vi "Temp_controller_with_cooling.vi"() -> ()   [LabVIEW 2017]
uses:
  <instrlib>/Lake Shore Cryotronics 332/Lake Shore Cryotronics 332.lvlib
panel:
  out "error out 2":errorcluster
  out "error out":errorcluster
  in  "Rate(D)":dbl min=0.0 max=200.0 step=1.0
  in  "Reset (I) (0.0)":dbl min=0.0 max=1000.0 step=0.1 format="%.1f"
  in  "Gain (P)":dbl min=0.0 max=1000.0 step=0.1 format="%.1f"
  in  "Manual Output":dbl min=0.0 max=100.0 step=0.001 format="%.3f"
  in  "Heater Range ()":u16(ring) items=["Off", "Low (0.5W)", "Med (5W)", "High (50W)"]
  out "Gain (P) 2":dbl min=0.0 max=1000.0 step=0.1 format="%.1f"
  out "Reset (I)":dbl min=0.0 max=1000.0 step=0.1 format="%.1f"
  out "Rate (D)":dbl min=0.0 max=1000.0 step=0.1 format="%.1f"
  out "Loop 1 Heater Range":u16(ring) items=["Off", "Low (0.5W)", "Med (5W)", "High (50W)"]
  in  "Enable Powerup ()":bool
  in  "Control Mode":u16(ring) items=["Manual PID", "Zone", "Open Loop", "AutoTune PID", "AutoTune PI", "AutoTune P"]
  out "return count 2":u32
  out "?":u32
  in  "error in (no error) 2":errorcluster
  in  "VISA resource name":refnum<visa-resource-name>
  in  "time interval to wait":dbl
  out "return count":u32
  out "?":u32
  in  "error in (no error)":errorcluster
  in  "Temo diff":dbl
  in  "End Temp":dbl
  in  "Start Temp":dbl
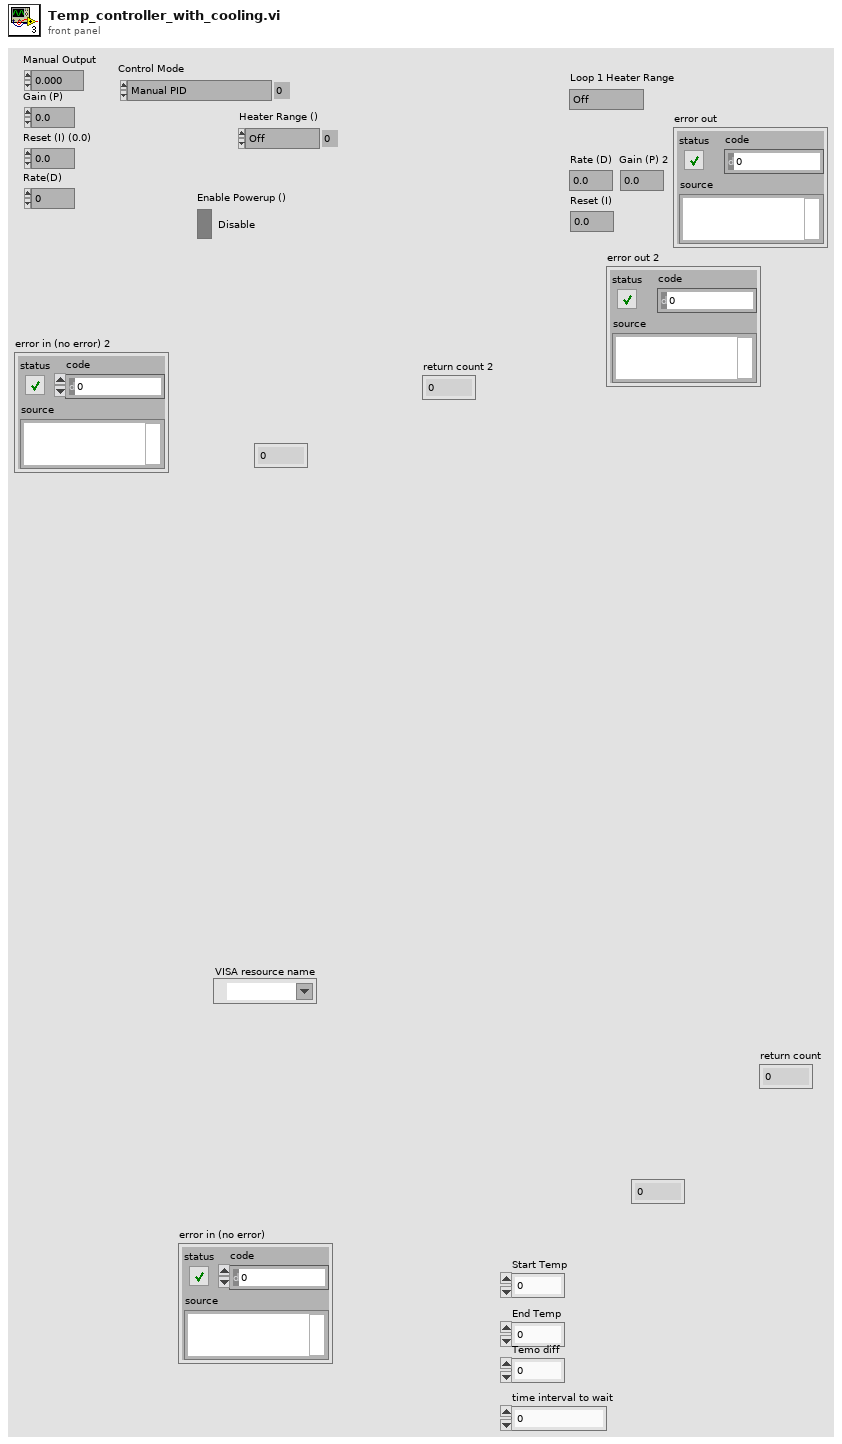
[diagram p1: front panel]
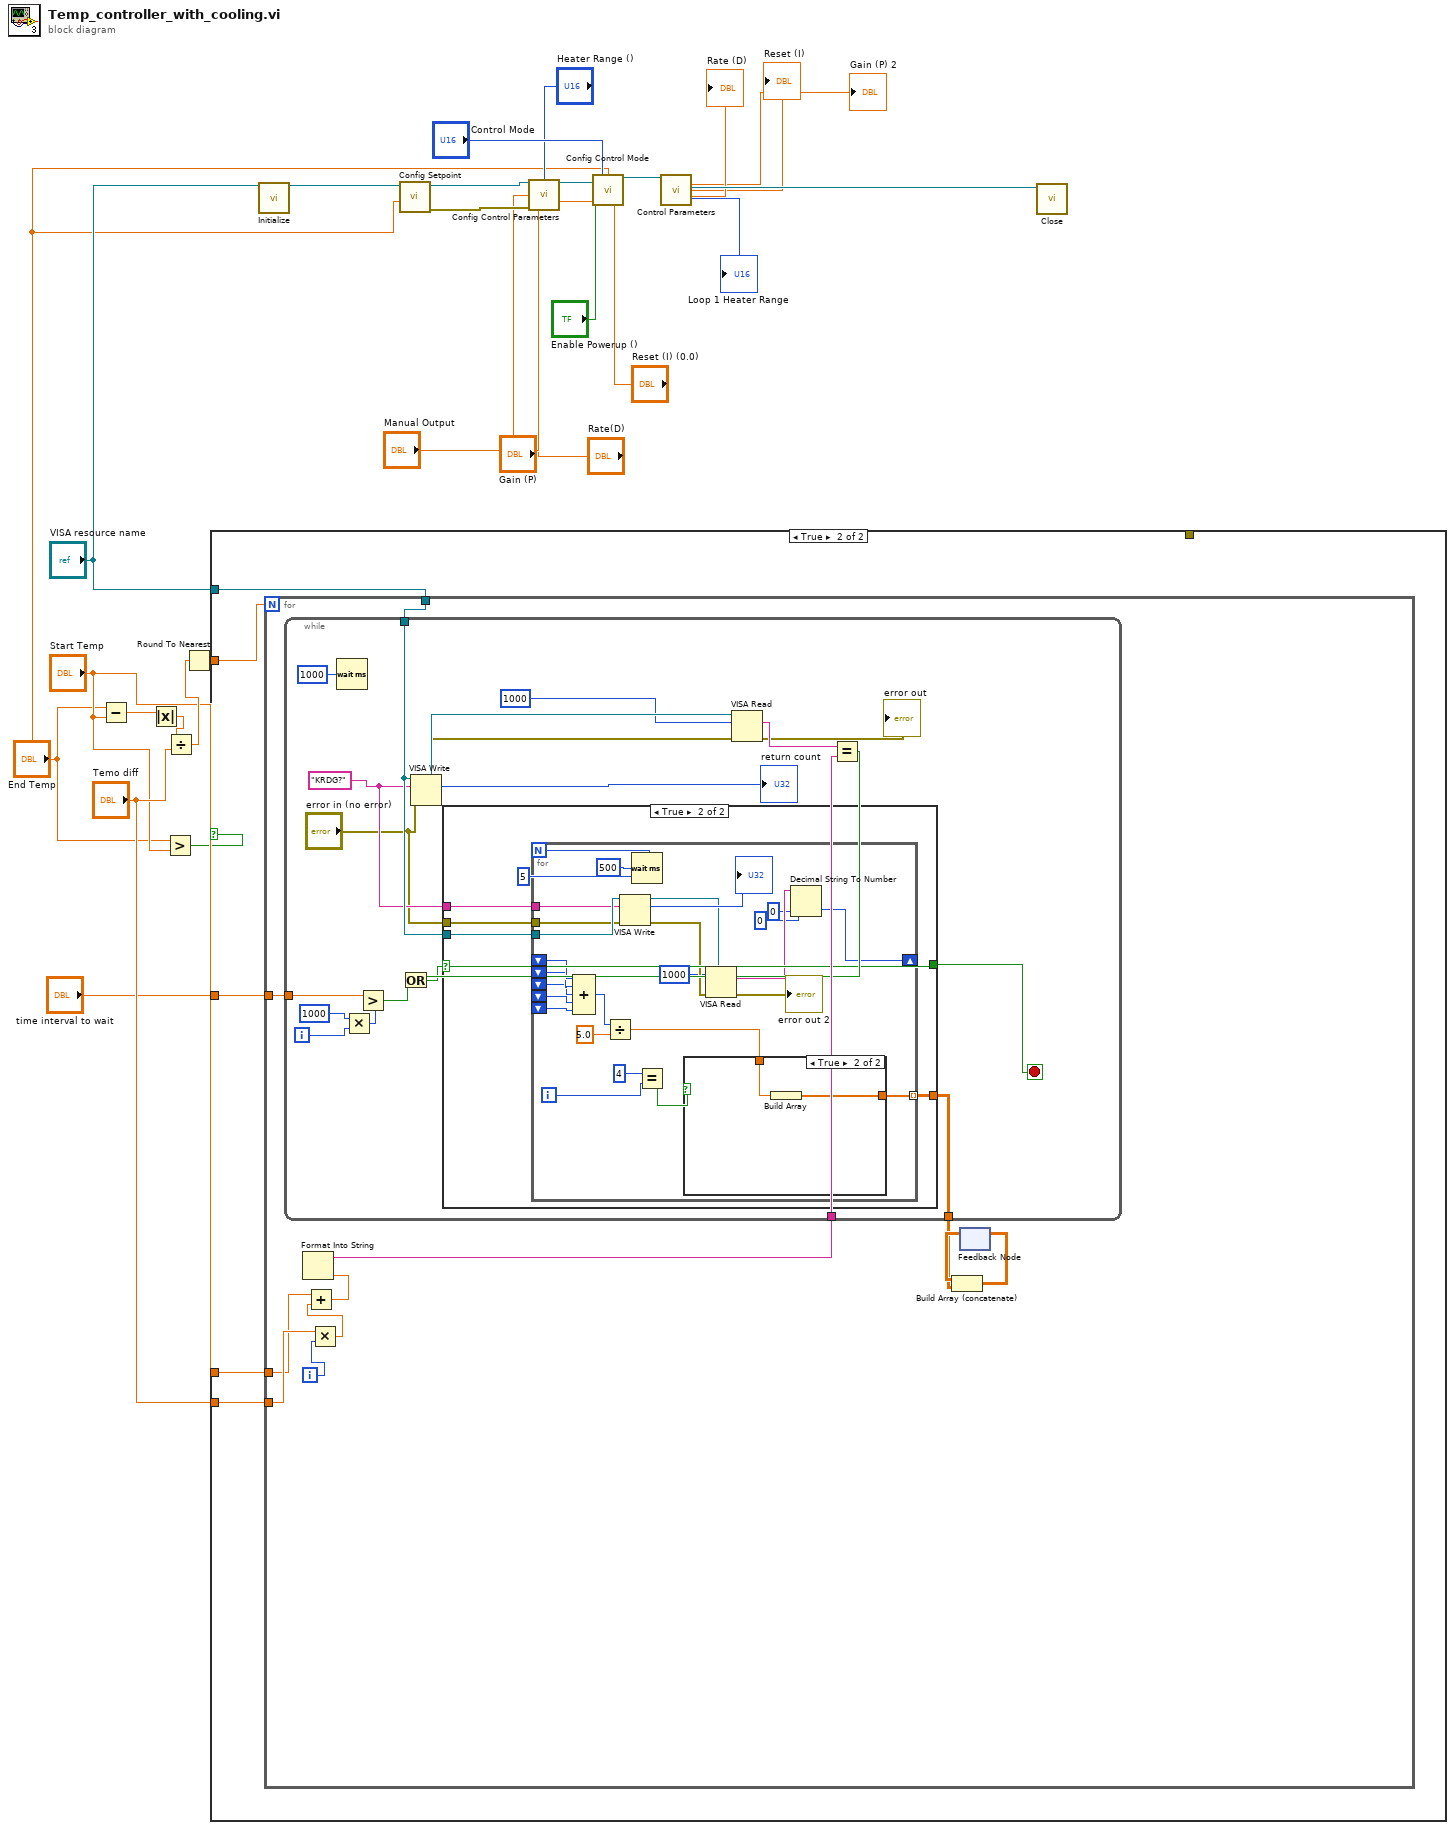
[diagram p0: block diagram]
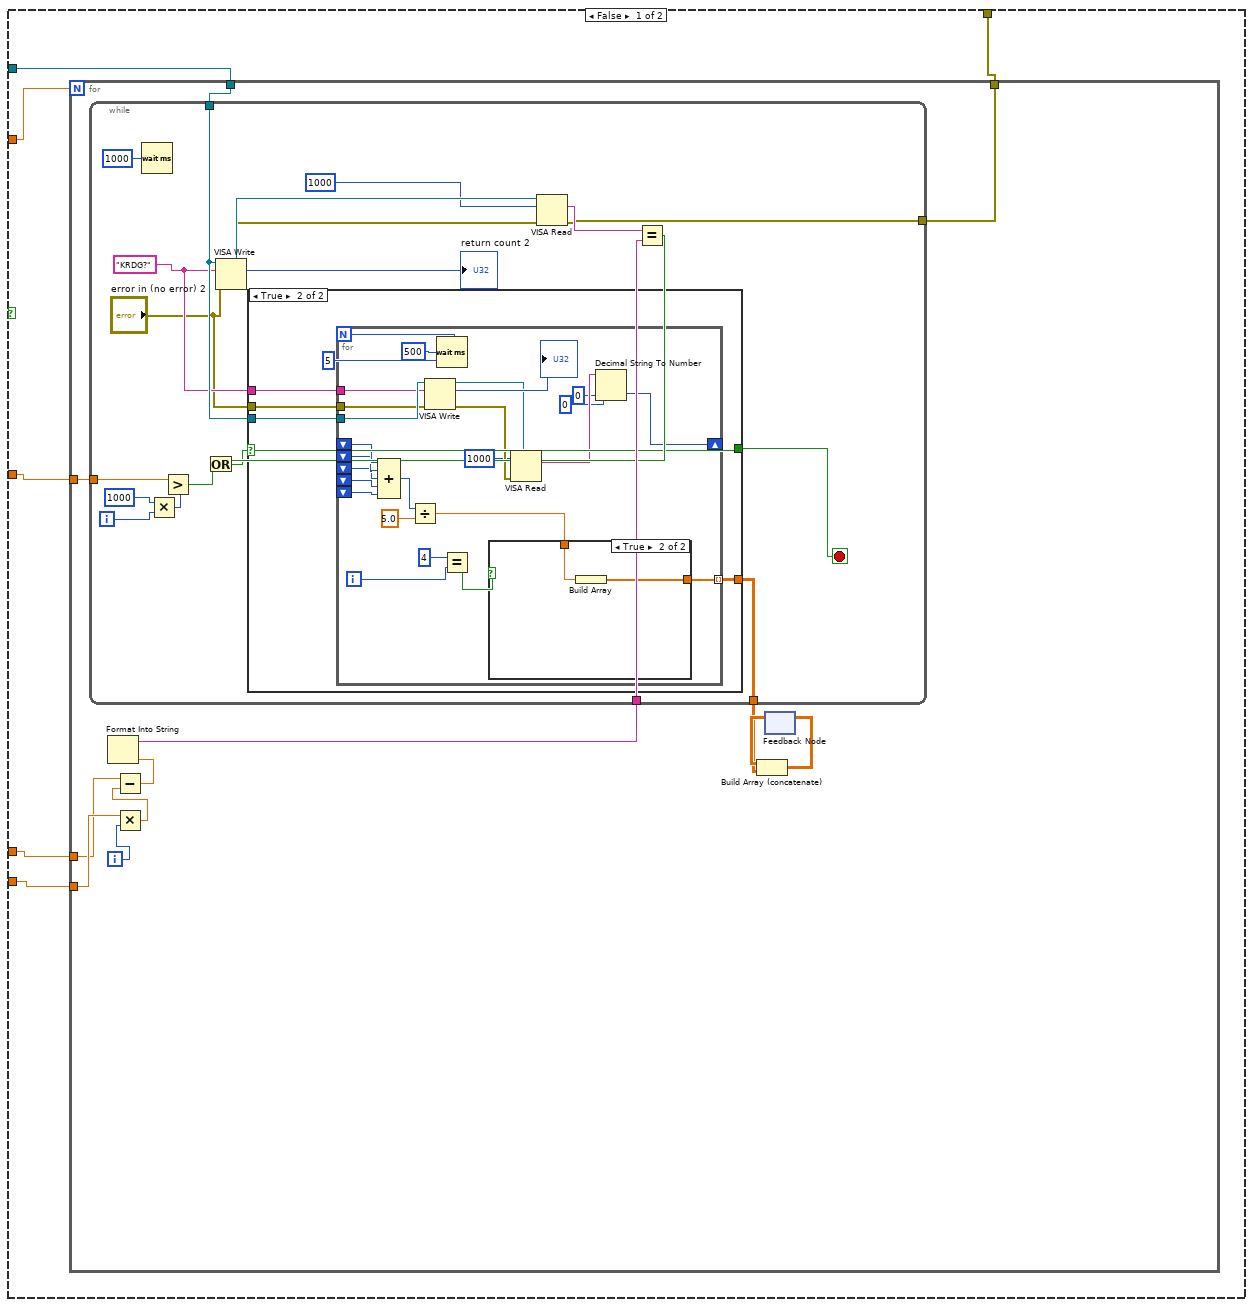
[diagram p2: hidden frame]
diagram:
  n1 = Subtract(x="End Temp", y="Start Temp") -> (x-y=w21:dbl)
  n2 = Absolute Value(x=w21) -> (abs(x)=w20:dbl)
  n3 = Greater?(x="End Temp", y="Start Temp") -> (0:w22:bool)
  n4 = Divide(x=w20, y="Temo diff") -> (x/y=w27:dbl)
  n5 = Round To Nearest(number=w27) -> (nearest integer value=w26:dbl)
  n6 = case shown="True" w22 {
    tunnel: w26 -> [w32 w103]
    tunnel: "Temo diff" -> [w28 w102]
    tunnel: "Start Temp" -> [w29 w101]
    tunnel: "VISA resource name" -> [w33 w100]
    tunnel: "time interval to wait" -> [w31 w99]
    tunnel: [w30 _] -> _
    frame False {
      n7 = for {
        N: w32 -> [_]
        tunnel: w28 -> [w45]
        tunnel: w29 -> [w36]
        tunnel: w33 -> [w44]
        tunnel: w31 -> [w43]
        tunnel: [w37] -> w30
        i -> [w42]
        n8 = Multiply(x=w45, y=w42) -> (x*y=w35:dbl)
        n9 = Subtract(x=w36, y=w35) -> (x-y=w34:dbl)
        n10 = Format Into String(w34) -> (resulting string=w41:string)  [unwired: 3 in, 1 out]
        n11 = while {
          tunnel: w44 -> [w54]
          tunnel: w41 -> [w60]
          tunnel: w43 -> [w55]
          tunnel: [w51] -> w38
          tunnel: [w46] -> w37
          i -> [w58]
          stop <- w48 stop-if-true
          w52 = "KRDG?" ("write buffer")
          n12 = Wait (ms)(milliseconds to wait=u32 1000) -> ()  [unwired: 1 out]
          n13 = Multiply(x=1000, y=w58) -> (x*y=w56:i32)
          n14 = Greater?(x=w55, y=w56) -> (0:w53:bool)
          n15 = VISA Write(VISA resource name=w54, write buffer=w52, error in (no error)="error in (no error) 2") -> (VISA resource name out=w64:refnum<visa-resource-name>, return count=→"return count 2":u32, error out=w62:errorcluster)
          n16 = VISA Read(VISA resource name=w64, byte count=u32 1000, error in (no error)=w62) -> (read buffer=w59:string, error out=w46:errorcluster)  [unwired: 2 out]
          n17 = Equal?(x=w59, y=w60) -> (x = y?=w50:bool)
          n18 = Or(x=w50, y=w53) -> (x .or. y?=w49:bool)
          n19 = case shown="True" w49 {
            selector: w49 -> [w66 w68]
            tunnel: w54 -> [_ w71]
            tunnel: w52 -> [_ w70]
            tunnel: [_ w69] -> w51
            tunnel: [w66 w68] -> w48
            tunnel: "error in (no error) 2" -> [_ w67]
            frame False {
            }
            frame True {
              n20 = for {
                N: 5 -> [_]
                tunnel: w71 -> [w93]
                shift-right: [w87] -> _
                shift-left: _ -> [w86]
                shift-left: _ -> [w85]
                shift-left: _ -> [w84]
                shift-left: _ -> [w83]
                shift-left: _ -> [w82]
                tunnel: w70 -> [w77]
                tunnel: [w75] -> w69 mode=indexing
                tunnel: w67 -> [w73]
                i -> [w79]
                n21 = Compound Arithmetic op=ADD(w86, w85, w84, w83, w82) -> (w80:i32)
                n22 = Divide(x=w80, y=5.0) -> (x/y=w76:dbl)
                n23 = VISA Write(VISA resource name=w93, write buffer=w77, error in (no error)=w73) -> (VISA resource name out=w92:refnum<visa-resource-name>, return count=→"?":u32, error out=w95:errorcluster)
                n24 = Wait (ms)(milliseconds to wait=u32 500) -> ()  [unwired: 1 out]
                n25 = Equal?(x=4, y=w79) -> (x = y?=w74:bool)
                n26 = case shown="True" w74 {
                  tunnel: w76 -> [_ w98]
                  tunnel: [_ w97] -> w75
                  frame False {
                  }
                  frame True {
                    n27 = Build Array(w98) -> (w97:dbl[])
                  }
                }
                n28 = VISA Read(VISA resource name=w92, byte count=u32 1000, error in (no error)=w95) -> (read buffer=w90:string)  [unwired: 3 out]
                n29 = Decimal String To Number(string=w90, offset=0, default (0L)=0 ("default (0 I32)")) -> (number=w87:i32)  [unwired: 1 out]
              }
            }
          }
        }
        n30 = feedback #1() -> (w39:dbl[][][])  [unwired: 1 in]
        n31 = Build Array (concatenate)(w39, w38) -> (w40:dbl[][][])
        n32 = feedback-in #1(w40) -> ()
      }
    }
    frame True {
      n33 = for {
        N: w103 -> [_]
        tunnel: w102 -> [w114]
        tunnel: w101 -> [w113]
        tunnel: w100 -> [w110]
        tunnel: w99 -> [w109]
        i -> [w108]
        n34 = Multiply(x=w114, y=w108) -> (x*y=w112:dbl)
        n35 = Add(x=w113, y=w112) -> (x+y=w111:dbl)
        n36 = Format Into String(w111) -> (resulting string=w107:string)  [unwired: 3 in, 1 out]
        n37 = while {
          tunnel: w110 -> [w123]
          tunnel: w107 -> [w129]
          tunnel: w109 -> [w124]
          tunnel: [w120] -> w104
          i -> [w127]
          stop <- w117 stop-if-true
          w121 = "KRDG?" ("write buffer")
          n38 = Wait (ms)(milliseconds to wait=u32 1000) -> ()  [unwired: 1 out]
          n39 = Multiply(x=1000, y=w127) -> (x*y=w125:i32)
          n40 = Greater?(x=w124, y=w125) -> (0:w122:bool)
          n41 = VISA Write(VISA resource name=w123, write buffer=w121, error in (no error)="error in (no error)") -> (VISA resource name out=w133:refnum<visa-resource-name>, return count=→"return count":u32, error out=w131:errorcluster)
          n42 = VISA Read(VISA resource name=w133, byte count=u32 1000, error in (no error)=w131) -> (read buffer=w128:string, error out=→"error out":errorcluster)  [unwired: 2 out]
          n43 = Equal?(x=w128, y=w129) -> (x = y?=w119:bool)
          n44 = Or(x=w119, y=w122) -> (x .or. y?=w118:bool)
          n45 = case shown="True" w118 {
            selector: w118 -> [w135 w137]
            tunnel: w123 -> [_ w140]
            tunnel: w121 -> [_ w139]
            tunnel: [_ w138] -> w120
            tunnel: [w135 w137] -> w117
            tunnel: "error in (no error)" -> [_ w136]
            frame False {
            }
            frame True {
              n46 = for {
                N: 5 -> [_]
                tunnel: w140 -> [w163]
                shift-right: [w157] -> _
                shift-left: _ -> [w156]
                shift-left: _ -> [w155]
                shift-left: _ -> [w154]
                shift-left: _ -> [w153]
                shift-left: _ -> [w152]
                tunnel: w139 -> [w147]
                tunnel: [w145] -> w138 mode=indexing
                tunnel: w136 -> [w143]
                i -> [w149]
                n47 = Compound Arithmetic op=ADD(w156, w155, w154, w153, w152) -> (w150:i32)
                n48 = Divide(x=w150, y=5.0) -> (x/y=w146:dbl)
                n49 = VISA Write(VISA resource name=w163, write buffer=w147, error in (no error)=w143) -> (VISA resource name out=w162:refnum<visa-resource-name>, return count=→"?":u32, error out=w165:errorcluster)
                n50 = Wait (ms)(milliseconds to wait=u32 500) -> ()  [unwired: 1 out]
                n51 = Equal?(x=4, y=w149) -> (x = y?=w144:bool)
                n52 = case shown="True" w144 {
                  tunnel: w146 -> [_ w168]
                  tunnel: [_ w167] -> w145
                  frame False {
                  }
                  frame True {
                    n53 = Build Array(w168) -> (w167:dbl[])
                  }
                }
                n54 = VISA Read(VISA resource name=w162, byte count=u32 1000, error in (no error)=w165) -> (read buffer=w160:string, error out=→"error out 2":errorcluster)  [unwired: 2 out]
                n55 = Decimal String To Number(string=w160, offset=0, default (0L)=0 ("default (0 I32)")) -> (number=w157:i32)  [unwired: 1 out]
              }
            }
          }
        }
        n56 = feedback #2() -> (w105:dbl[][][])  [unwired: 1 in]
        n57 = Build Array (concatenate)(w105, w104) -> (w106:dbl[][][])
        n58 = feedback-in #2(w106) -> ()
      }
    }
  }
  n59 = call <instrlib>:"Initialize.vi"("VISA resource name"="VISA resource name") -> ("VISA resource name out"=w19:refnum<visa-resource-name>)  [unwired: 13 in, 1 out]
  n60 = call <instrlib>:"Config Setpoint.vi"("Setpoint (0.0000)"="End Temp", "VISA resource name"=w19) -> ("error out"=w10:errorcluster, "VISA resource name out"=w11:refnum<visa-resource-name>)  [unwired: 8 in]
  n61 = call <instrlib>:"Config Control Parameters.vi"("VISA resource name"=w11, "Manual Output (0.000)"="Manual Output", "Heater Range (0: Off)"="Heater Range ()", "Gain (P) (0.0)"="Gain (P)", "Reset (I) (0.0)"="Reset (I) (0.0)", "error in (no error)"=w10, "Rate (D) (0)"="Rate(D)") -> ("VISA resource name out"=w9:refnum<visa-resource-name>)  [unwired: 7 in, 1 out]
  n62 = call <instrlib>:"Config Control Mode.vi"("VISA resource name"=w9, "Control Mode (0: Manual PID)"="Control Mode", "Setpoint Units (0: Kelvin)"="End Temp", "Enable Powerup (F: Enable)"="Enable Powerup ()") -> ("VISA resource name out"=w3:refnum<visa-resource-name>)  [unwired: 10 in, 1 out]
  n63 = call <instrlib>:"Control Parameters.vi"("VISA resource name"=w3) -> ("VISA resource name out"=w18:refnum<visa-resource-name>, "Gain (P)"=→"Gain (P) 2":dbl, "Reset (I)"=→"Reset (I)":dbl, "Rate (D)"=→"Rate (D)":dbl, "Loop 1 Heater Range"=→"Loop 1 Heater Range":u16)  [unwired: 7 in, 3 out]
  n64 = call <instrlib>:"Close.vi"("VISA resource name"=w18) -> ()  [unwired: 10 in, 1 out]
